vi "unescape json string.vi"(9 "quotes removed?":bool, 11 "base string":string) -> (3 "String out":string)   [LabVIEW 2013, in "json generator.lvlib"]
uses:
  json generator.lvlib
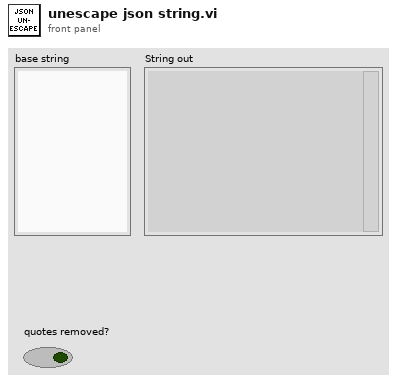
[diagram p1: front panel]
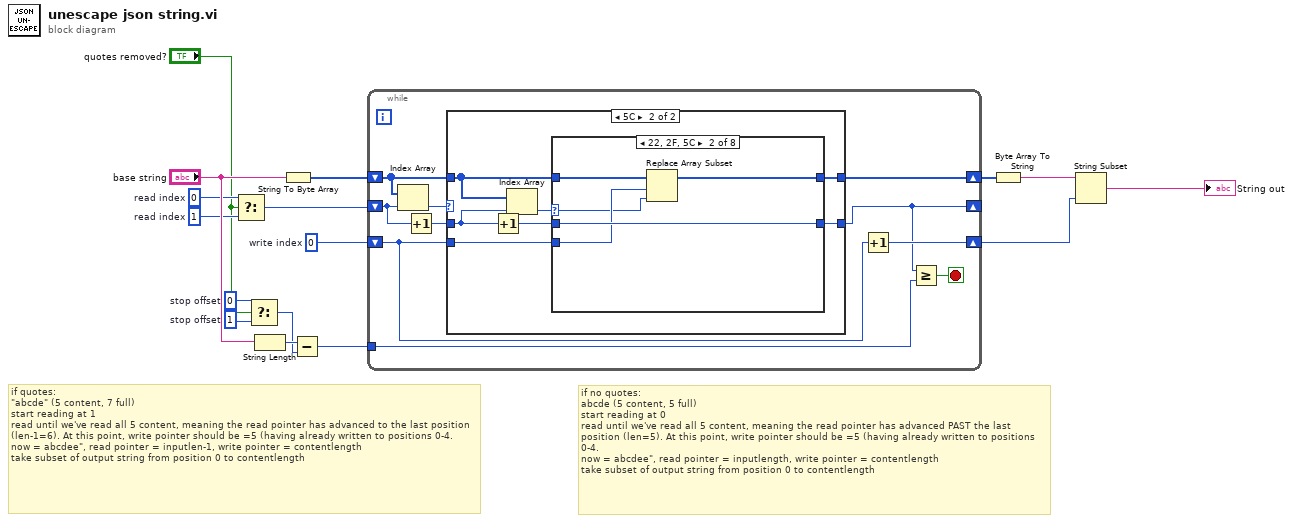
[diagram p0: block diagram]
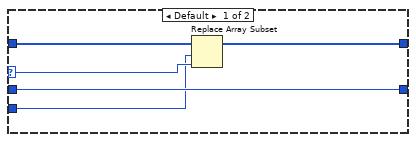
[diagram p2: hidden frame]
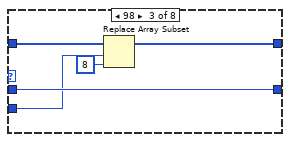
[diagram p4: hidden frame]
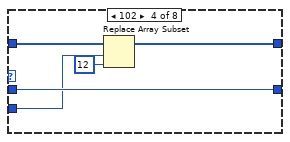
[diagram p5: hidden frame]
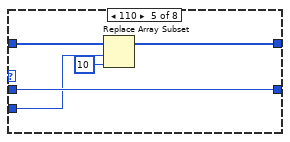
[diagram p6: hidden frame]
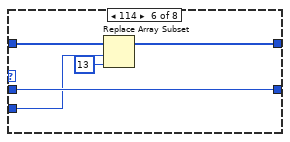
[diagram p7: hidden frame]
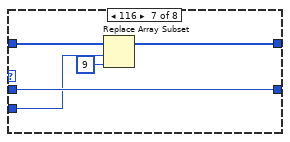
[diagram p8: hidden frame]
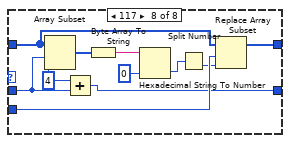
[diagram p9: hidden frame]
diagram:
  w4 = 0  # stop offset
  w3 = 1  # stop offset
  w9 = 0  # read index
  w8 = 1  # read index
  w12 = 0  # write index
  # "if no quotes:\nabcde (5 content, 5 full)\nstart reading at 0\nread until we've read all 5 content, meaning the read pointer has advanced PAST the last position (len=5). At this point, write pointer should be =5 (having already written to positions 0-4.\nnow = abcdee\", read pointer = inputlength, write pointer = contentlength\ntake subset of output string from position 0 to contentlength"
  # "if quotes:\n\"abcde\" (5 content, 7 full)\nstart reading at 1\nread until we've read all 5 content, meaning the read pointer has advanced to the last position (len-1=6). At this point, write pointer should be =5 (having already written to positions 0-4.\nnow = abcdee\", read pointer = inputlen-1, write pointer = contentlength\ntake subset of output string from position 0 to contentlength"
  n1 = Select(t=w9, s="quotes removed?", f=w8) -> (s? t:f=w7:i32)
  n2 = Select(t=w4, s="quotes removed?", f=w3) -> (s? t:f=w1:i32)
  n3 = String Length(string="base string") -> (length=w2:i32)
  n4 = String To Byte Array(string="base string") -> (unsigned byte array=w14:u8[])
  n5 = Subtract(x=w2, y=w1) -> (x-y=w10:i32)
  n6 = while {
    shift-right: [w24] -> w11
    shift-left: w14 -> [w25]
    shift-right: [w17] -> _
    shift-left: w7 -> [w21]
    shift-right: [w18] -> w6
    shift-left: w12 -> [w22]
    tunnel: w10 -> [w19]
    stop <- w20 stop-if-true
    n7 = Index Array(array=w25, index=w21) -> (element=w26:u8)
    n8 = Increment(x=w21) -> (x+1=w23:i32)
    n9 = case shown="5C" w26 {
      selector: w26 -> [w28 _]
      tunnel: w25 -> [w31 w37]
      tunnel: [w29 w36] -> w24
      tunnel: w23 -> [w30 w34]
      tunnel: w22 -> [w27 w35]
      tunnel: [w30 w33] -> w17
      frame Default {
        n10 = Replace Array Subset(array=w31, new element=w28, index=w27) -> (w29:u8[])
      }
      frame 92 {
        n11 = Increment(x=w34) -> (x+1=w32:i32)
        n12 = Index Array(array=w37, index=w34) -> (element=w38:u8)
        n13 = case shown="22, 2F, 5C" w38 {
          selector: w38 -> [_ w41 _ _ _ _ _ _]
          tunnel: w37 -> [w40 w45 w50 w55 w60 w65 w70 w78]
          tunnel: [w40 w44 w49 w54 w59 w64 w69 w79] -> w36
          tunnel: w35 -> [_ w42 w47 w52 w57 w62 w67 w77]
          tunnel: w32 -> [w39 w43 w48 w53 w58 w63 w68 w80]
          tunnel: [w39 w43 w48 w53 w58 w63 w68 w76] -> w33
          frame Default {
            # "error"
          }
          frame 34, 47, 92 {
            n14 = Replace Array Subset(array=w45, new element=w41, index=w42) -> (w44:u8[])
          }
          frame 98 {
            n15 = Replace Array Subset(array=w50, new element=u8 8 ("new element/subarray"), index=w47) -> (w49:u8[])
          }
          frame 102 {
            n16 = Replace Array Subset(array=w55, new element=u8 12 ("new element/subarray"), index=w52) -> (w54:u8[])
          }
          frame 110 {
            n17 = Replace Array Subset(array=w60, new element=u8 10 ("new element/subarray"), index=w57) -> (w59:u8[])
          }
          frame 114 {
            n18 = Replace Array Subset(array=w65, new element=u8 13 ("new element/subarray"), index=w62) -> (w64:u8[])
          }
          frame 116 {
            n19 = Replace Array Subset(array=w70, new element=u8 9 ("new element/subarray"), index=w67) -> (w69:u8[])
          }
          frame 117 {
            w81 = 4 ("length")
            n20 = Array Subset(array=w78, index=w80, length=w81) -> (w75:u8[])
            n21 = Add(x=w81, y=w80) -> (x+y=w76:i32)
            n22 = Byte Array To String(unsigned byte array=w75) -> (string=w74:string)
            n23 = Hexadecimal String To Number(string=w74, default (0uL)=u16 0 ("default (0 U32)")) -> (number=w72:u16)  [unwired: 1 in, 1 out]
            n24 = Split Number(x=w72) -> (lo(x)=w71:u8)  [unwired: 1 out]
            n25 = Replace Array Subset(array=w78, new element=w71, index=w77) -> (w79:u8[])
          }
        }
      }
    }
    n26 = Increment(x=w22) -> (x+1=w18:i32)
    n27 = Greater Or Equal?(x=w17, y=w19) -> (x >= y?=w20:bool)
  }
  n28 = Byte Array To String(unsigned byte array=w11) -> (string=w13:string)
  n29 = String Subset(string=w13, length (rest)=w6) -> (substring=→"String out":string)  [unwired: 1 in]
